vi "Check System Readiness.vi"(8 "error in (no error)":errorcluster) -> (0 "error out":errorcluster, 3 "Readiness Check Results":T1[](array[typedef]))   [LabVIEW 2026, in "Framework Engine.lvclass"]
uses:
  Framework Engine.lvclass
  Framework Engine.lvclass/Framework Engine.ctl
  Services/Readiness Service/Readines Service.lvclass
  Typedefs/enums/Readiness State Enum.ctl
  Typedefs/clusters/Readiness Check Result.ctl
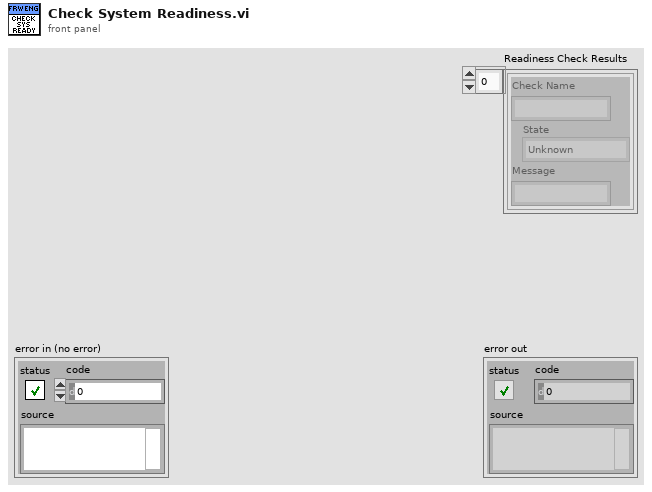
[diagram p1: front panel]
types:
  T1 = typedef "Readiness Check Result.ctl" = cluster{"Check Name":string, "State":T2, "Message":string}
  T2 = typedef "Readiness State Enum.ctl" = enum16{"Unknown", "Ready", "Warning", "NotReady"}
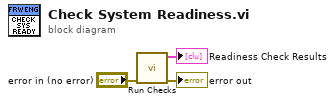
[diagram p0: block diagram]
diagram:
  n1 = call "Run Checks.vi"("error in (no error)"="error in (no error)") -> ("error out"=→"error out":errorcluster, "Readiness Check Results"=→"Readiness Check Results":T1[])  [unwired: 9 in]
